vi "Compare ECAT FPGA Wrapper.vi"(8 "error in (no error)":errorcluster, 10 "UDV Container in":refnum<k21>, 11 "FPGA in":T1 {"UDVs"."To FPGA"."VS ref" format="%.0x"; "UDVs"."From FPGA"."VS ref" format="%.0x"; "VS ref" format="%.0x"; "Output Data"."BD Refs"."Data Reference" format="%.0x"; "Input Data"."BD Refs"."Data Reference" format="%.0x"}) -> (0 "error out":errorcluster, 1 "Same?":bool, 2 "UDV Container out":refnum<k21>, 3 "FPGA out":T1 {"UDVs"."To FPGA"."VS ref" format="%.0x"; "UDVs"."From FPGA"."VS ref" format="%.0x"; "VS ref" format="%.0x"; "Output Data"."BD Refs"."Data Reference" format="%.0x"; "Input Data"."BD Refs"."Data Reference" format="%.0x"})   [LabVIEW 2016, in "Scan Engine Custom Device.lvlib"]
uses:
  Scan Engine Custom Device.lvlib
  Type Defs/FPGA Data.ctl
  <vilib>/NI Veristand/Custom Device API/Custom Device Item Ref.ctl
  Type Defs/Input Data.ctl
  <vilib>/NI Veristand/Custom Device API/Block Data Reference.ctl
  <vilib>/NI Veristand/Custom Device API/Data Reference.ctl
  Type Defs/Output Data.ctl
  Type Defs/UDV Data.ctl
  Type Defs/UDV Data Type.ctl
  Type Defs/FXP Config.ctl
  <vilib>/NI Veristand/Custom Device API/Custom Device API.lvlib
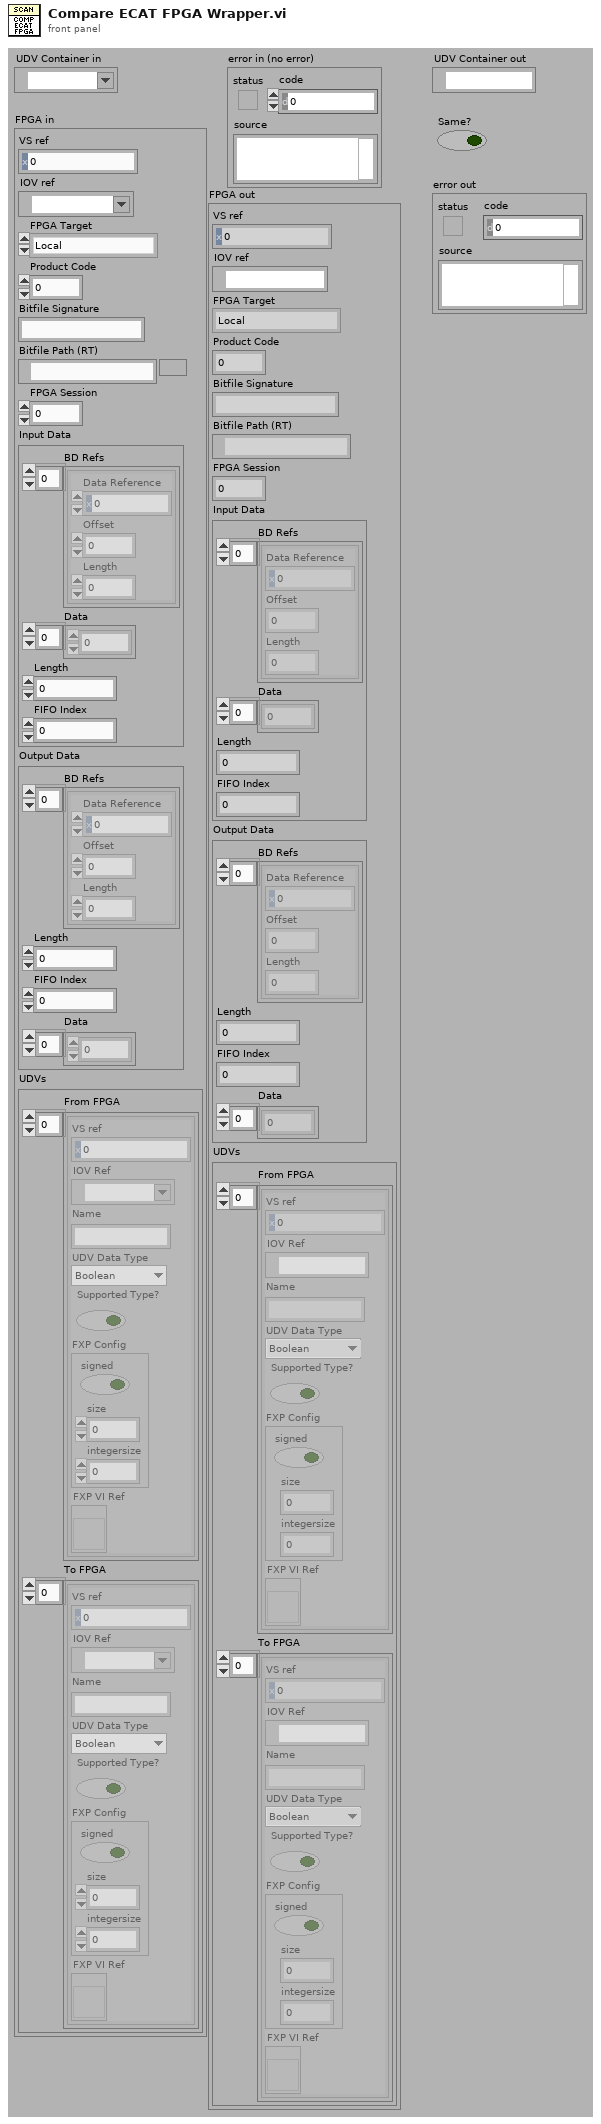
[diagram p1: front panel]
types:
  T1 = typedef "Scan Engine Custom Device.lvlib/FPGA Data.ctl" = cluster{"VS ref":T2, "IOV ref":refnum<k21>, "FPGA Target":enum16{"Local", "EtherCAT"}, "Product Code":u32, "Bitfile Signature":string, "Bitfile Path (RT)":path, "FPGA Session":u32, "Input Data":T3, "Output Data":T6, "UDVs":cluster{"From FPGA":T7[], "To FPGA":T7[]}}
  T2 = typedef "Custom Device API.lvlib/Custom Device Item Ref.ctl" = u64
  T3 = typedef "Scan Engine Custom Device.lvlib/Input Data.ctl" = cluster{"BD Refs":T4[], "Data":dbl[], "Length":i32, "FIFO Index":i32}
  T4 = typedef "Custom Device API.lvlib/Block Data Reference.ctl" = cluster{"Data Reference":T5, "Offset":u64, "Length":u64}
  T5 = typedef "Custom Device API.lvlib/Data Reference.ctl" = i32
  T6 = typedef "Scan Engine Custom Device.lvlib/Output Data.ctl" = cluster{"BD Refs":T4[], "Length":i32, "FIFO Index":i32, "Data":dbl[]}
  T7 = typedef "Scan Engine Custom Device.lvlib/UDV Data.ctl" = cluster{"VS ref":T2, "IOV Ref":refnum<k21>, "Name":string, "UDV Data Type":T8, "Supported Type?":bool, "FXP Config":T9, "FXP VI Ref":refnum<vi>}
  T8 = typedef "Scan Engine Custom Device.lvlib/UDV Data Type.ctl" = enum16{"Boolean", "Fixed Point", "Int8", "Int16", "Int32", "Int64", "U32 Bit Field", "UInt8", "UInt16", "UInt32", "UInt64", "Other"}
  T9 = typedef "Scan Engine Custom Device.lvlib/FXP Config.ctl" = cluster{"signed":bool, "size":u32, "integersize":i32}
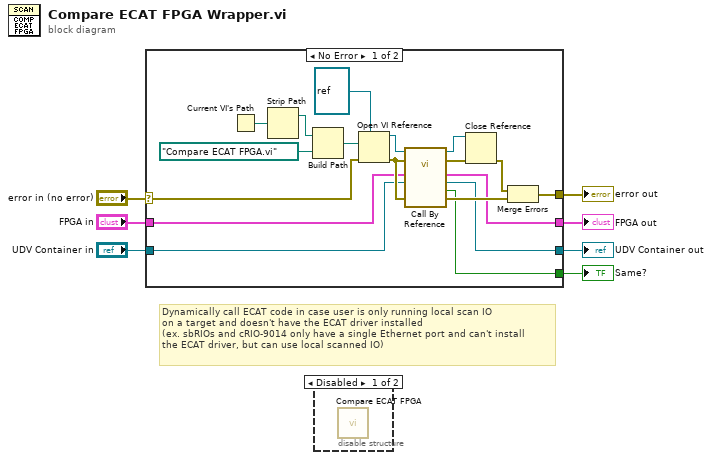
[diagram p0: block diagram]
diagram:
  # "Dynamically call ECAT code in case user is only running local scan IO\non a target and doesn't have the ECAT driver installed\n(ex. sbRIOs and cRIO-9014 only have a single Ethernet port and can't install\nthe ECAT driver, but can use local scanned IO)"
  n1 = case shown="No Error" "error in (no error)" {
    selector: "error in (no error)" -> [w15 w27]
    tunnel: [w10 w28] -> w7
    tunnel: [w14 w27] -> w6
    tunnel: "UDV Container in" -> [w12 w28]
    tunnel: [w9 _] -> w4
    tunnel: "FPGA in" -> [w13 w26]
    tunnel: [w11 w26] -> w1
    frame No Error {
      n2 = Current VI's Path() -> (path=w25:path)
      n3 = Strip Path(path=w25) -> (stripped path=w23:path)  [unwired: 1 out]
      n4 = Build Path(base path=w23, name or relative path=path "Compare ECAT FPGA.vi" ("vi path")) -> (appended path=w22:path)
      n5 = Open VI Reference(type specifier VI Refnum (for type only)=refnum<vi> refnum, vi path=w22, error in (no error)=w15) -> (vi reference=w20:refnum<vi>, error out=w21:errorcluster)  [unwired: 3 in]
      n6 = call-by-ref "?"(reference=w20, error in=w21, 8:"error in (no error)"=w21, "UDV Container in"=w12, "FPGA in"=w13) -> (reference out=w18:refnum<vi>, error out=w19:errorcluster, 0:"error out"=w17:errorcluster, "Same?"=w9:bool, "UDV Container out"=w10:refnum<k21>, "FPGA out"=w11:T1)  [unwired: 5 in]
      n7 = Close Reference(reference=w18, error in (no error)=w19) -> (error out=w16:errorcluster)
      n8 = Merge Errors(w16, w17) -> (w14:errorcluster)
    }
    frame Error {
    }
  }
  "UDV Container out" <- w7
  "error out" <- w6
  "Same?" <- w4
  "FPGA out" <- w1
  n9 = disable-structure shown="Disabled" {
    frame Disabled {
      n10 = call "Compare ECAT FPGA.vi"() -> ()  [unwired: 8 in, 4 out]
    }
    frame Enabled {
    }
  }
